vi "Write Y_preSet.vi"(10 "Y_preSet":dbl, 11 "reg in":refnum<class "bronkhorst_reg_2.lvclass">) -> (3 "reg out":refnum<class "bronkhorst_reg_2.lvclass">)   [LabVIEW 2019, in "control.lvlib" / "bronkhorst_reg_2.lvclass"]
uses:
  bronkhorst_reg_2.lvclass
  bronkhorst_reg_2.lvclass/bronkhorst_reg_2.ctl
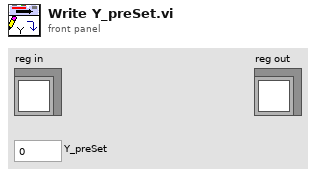
[diagram p1: front panel]
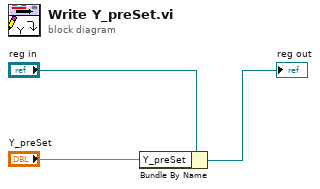
[diagram p0: block diagram]
diagram:
  n1 = Bundle By Name(cluster="reg in", "Y_preSet"="Y_preSet") -> (→"reg out":refnum<class "bronkhorst_reg_2.lvclass">)
